vi "ConnectToVLCPlayer.vi"(8 "error in":errorcluster, 10 "VLC Port":u16=65123, 11 "VLC IP address":string="127.0.0.1") -> (0 "error out":errorcluster, 3 "Connection ID":refnum<k5>)   [LabVIEW 2015]
doc: "Low level VI for connecting to an open VLC interface. Generally don't use this, use \"OpenVLCPlayer\" instead."
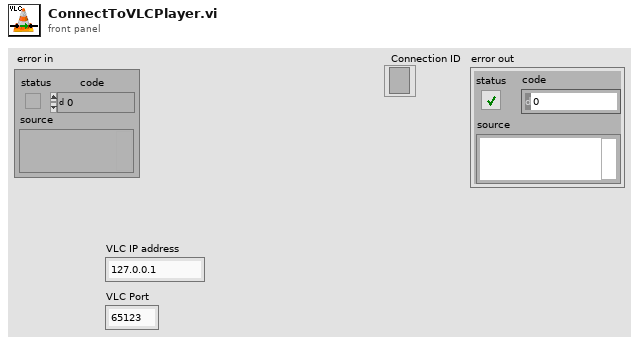
[diagram p1: front panel]
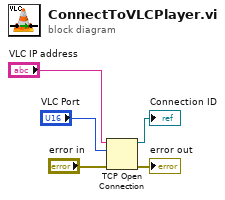
[diagram p0: block diagram]
diagram:
  n1 = TCP Open Connection(address="VLC IP address", remote port or service name="VLC Port", error in (no error)="error in") -> (connection ID=→"Connection ID":refnum<k5>, error out=→"error out":errorcluster)  [unwired: 2 in]
